vi "Host - Update Stop.vi"(6 "Operation":enum16{"Init", "Get", "Set"}(ring)=enum."Get", 8 "error in":errorcluster, 10 "Stop in":bool) -> (0 "error out":errorcluster, 2 "Stop?":bool)   [LabVIEW 2021]
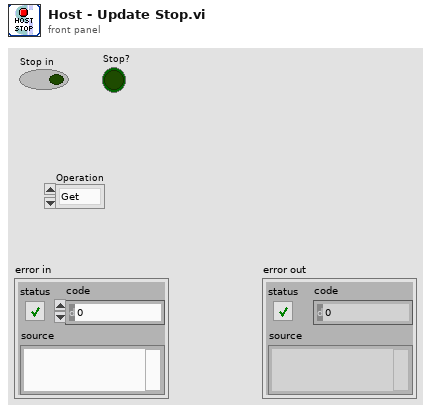
[diagram p1: front panel]
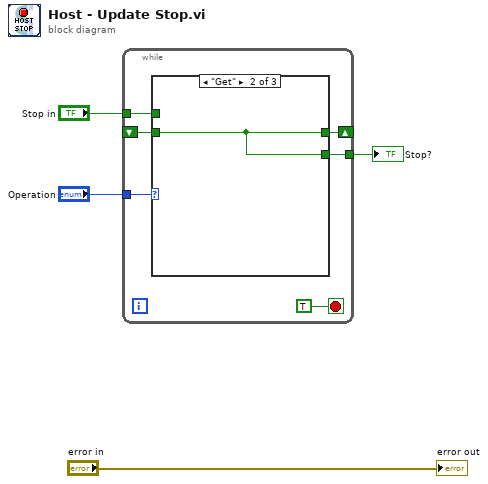
[diagram p0: block diagram]
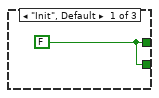
[diagram p2: hidden frame]
diagram:
  n1 = while {
    tunnel: "Operation" -> [w9]
    shift-right: [w8] -> _
    shift-left: _ -> [w7]
    tunnel: [w6] -> w3
    tunnel: "Stop in" -> [w5]
    stop <- TRUE stop-if-true
    n2 = case shown="\"Get\"" w9 {
      tunnel: [w11 w12 w13] -> w8
      tunnel: w7 -> [_ w12 _]
      tunnel: [w11 w12 w13] -> w6
      tunnel: w5 -> [_ _ w13]
      frame "Init", Default {
        w11 = FALSE
      }
      frame "Get" {
      }
      frame "Set" {
      }
    }
  }
  "Stop?" <- w3
  "error out" <- "error in"
